vi "dataSave.vi"(8 "error in (no error)":errorcluster) -> (0 "error out":errorcluster)   [LabVIEW 2019]
uses:
  _ctrl/create-rw-close.ctl
  _ctrl/init-r-stop.ctl
  type-data.ctl
  _ctrl/rw.ctl
panel:
  out "# elements in queue":i32
  out "Numeric":i32
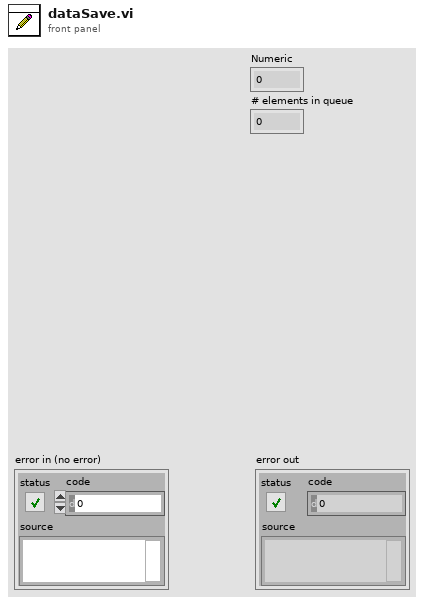
[diagram p1: front panel]
types:
  T1 = typedef "create-rw-close.ctl" = enum16{"create", "write", "read", "delete", "close"}
  T2 = typedef "init-r-stop.ctl" = enum16{"ini", "read", "stop"}
  T3 = typedef "type-data.ctl" = cluster{"dup path":path, "data":string}
  T4 = enum16{"open", "replace", "create", "open or create", "replace or create", "replace or create with confirmation"}
  T5 = typedef "rw.ctl" = enum16{"read", "write"}
  T6 = typedef "config_aging.ctl" = cluster{"Setting":T7, "TestName":string, "Result path":path, "파일 생성 주기[N]":u8, "Test Specs":T8}
  T7 = typedef "Setting_reg.ctl" = cluster{"제어 전압[V]":dbl, "출력전압[V]":dbl, "전류[A]":dbl, "출력전류[A]":dbl, "ON[초]":dbl, "OFF[초]":dbl, "Irms 허용치 from ":dbl, "Irms 허용치 to":dbl, "AO Delay ms":u32, "Log":path, "result":path}
  T8 = typedef "Breakdown-Spec.ctl" = cluster{"제어단 단선 Irms[mA](이하)":dbl, "제어단 특성 전류 Irms[mA] Max":dbl, "제어단 특성 전류 Irms[mA] Min":dbl, "출력단 단선 Irms[mA](이하)":dbl, "출력단 특성 전류 Irms[mA]  Max":dbl, "출력단 특성전류 Irms[mA]  Min":dbl, "온도[degree]":dbl}
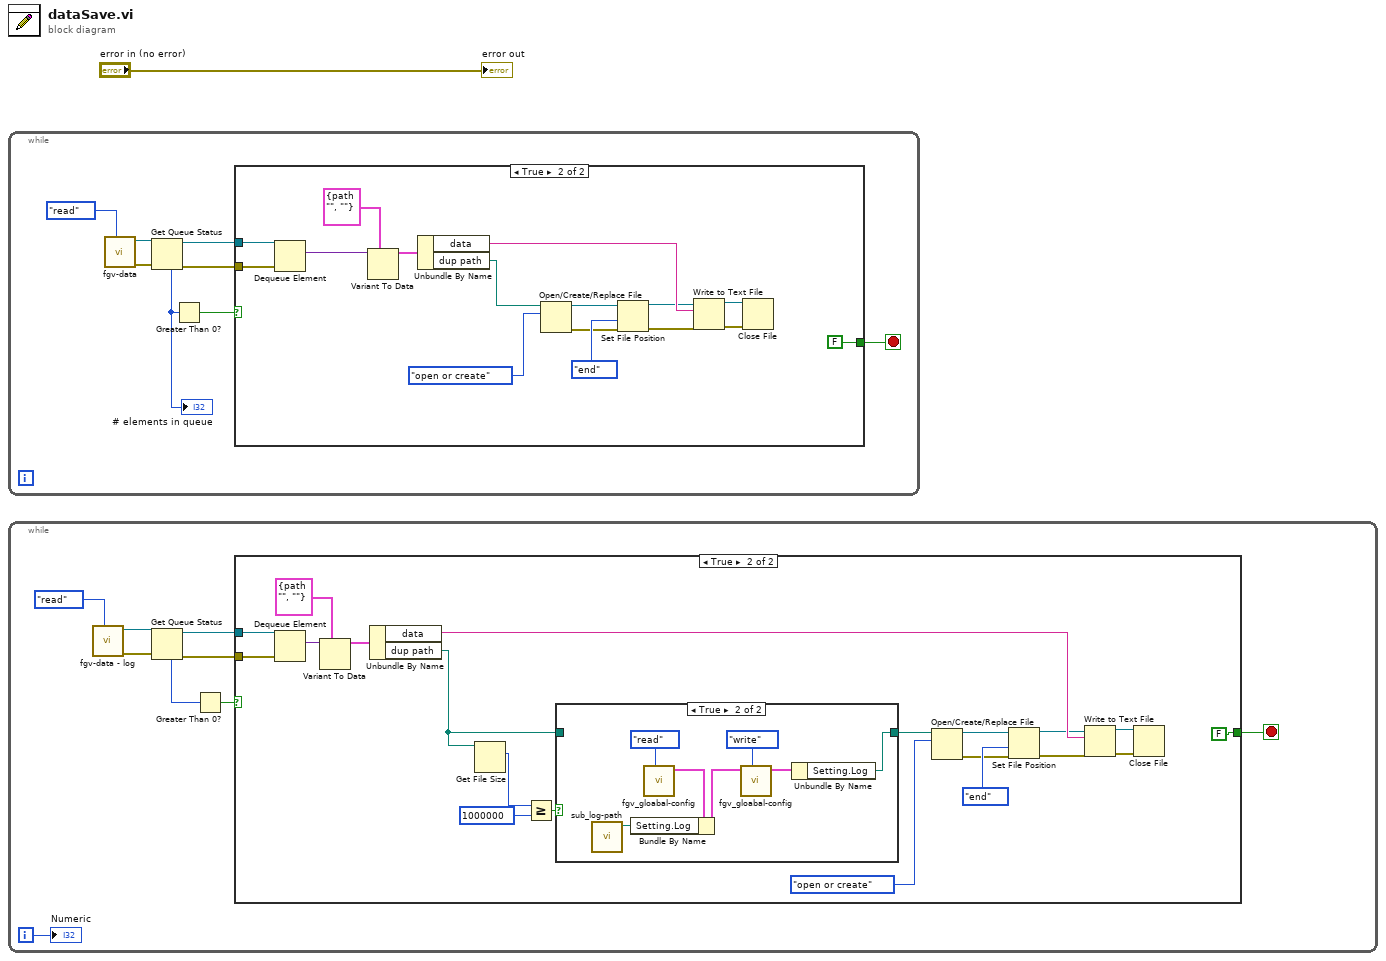
[diagram p0: block diagram]
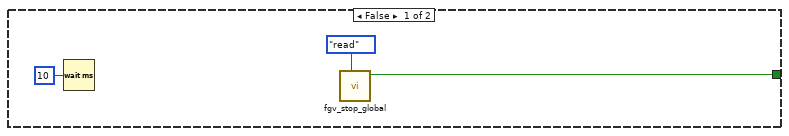
[diagram p2: hidden frame]
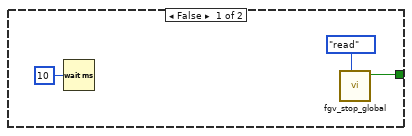
[diagram p4: hidden frame]
diagram:
  n1 = while {
    stop <- w3 stop-if-true
    n2 = call "fgv-data.vi"("cmd"=create-rw-close."read") -> ("error out"=w7:errorcluster, "queue out"=w8:refnum<queue>)  [unwired: 9 in]
    n3 = Get Queue Status(queue=w8, error in (no error)=w7) -> (queue out=w5:refnum<queue>, error out=w4:errorcluster, # elements in queue=w6:i32)  [unwired: 1 in, 5 out]
    "# elements in queue" <- w6
    n4 = Greater Than 0?(x=w6) -> (x > 0?=w2:bool)
    n5 = case shown="True" w2 {
      tunnel: w5 -> [_ w28]
      tunnel: w4 -> [_ w27]
      tunnel: [w11 FALSE] -> w3
      frame False {
        n6 = Wait (ms)(milliseconds to wait=u32 10) -> ()  [unwired: 1 out]
        n7 = call "fgv_stop_global.vi"("cmd"=init-r-stop."read") -> ("stop"=w11:bool)  [unwired: 10 in]
      }
      frame True {
        n8 = Dequeue Element(queue=w28, error in (no error)=w27) -> (element=w22:variant)  [unwired: 1 in, 3 out]
        n9 = Variant To Data(type=T3 {"dup path"=path "", "data"=""}, Variant=w22) -> (data=w20:T3)  [unwired: 1 in, 1 out]
        n10 = Unbundle By Name(w20) -> ("data"=w18:string, "dup path"=w19:path)
        n11 = Open/Create/Replace File(file path (use dialog)=w19, operation (0:open)=T4."open or create") -> (refnum out=w16:refnum<file>, error out=w14:errorcluster)  [unwired: 4 in, 1 out]
        n12 = Set File Position(refnum=w16, from (0:start)=enum16{"start", "end", "current"}."end", error in=w14) -> (refnum out=w15:refnum<file>, error out=w13:errorcluster)  [unwired: 1 in]
        n13 = Write to Text File(file (use dialog)=w15, text=w18, error in=w13) -> (refnum out=w25:refnum<file>, error out=w24:errorcluster)  [unwired: 1 in, 1 out]
        n14 = Close File(refnum=w25, error in=w24) -> ()  [unwired: 2 out]
      }
    }
  }
  n15 = while {
    i -> [w29]
    stop <- w34 stop-if-true
    n16 = call "fgv-data - log.vi"("cmd"=create-rw-close."read") -> ("error out"=w31:errorcluster, "queue out"=w32:refnum<queue>)  [unwired: 9 in]
    n17 = Get Queue Status(queue=w32, error in (no error)=w31) -> (queue out=w36:refnum<queue>, error out=w35:errorcluster, # elements in queue=w37:i32)  [unwired: 1 in, 5 out]
    n18 = Greater Than 0?(x=w37) -> (x > 0?=w30:bool)
    n19 = case shown="True" w30 {
      tunnel: w36 -> [_ w60]
      tunnel: w35 -> [_ w59]
      tunnel: [w39 FALSE] -> w34
      frame False {
        n20 = Wait (ms)(milliseconds to wait=u32 10) -> ()  [unwired: 1 out]
        n21 = call "fgv_stop_global.vi"("cmd"=init-r-stop."read") -> ("stop"=w39:bool)  [unwired: 10 in]
      }
      frame True {
        n22 = Dequeue Element(queue=w60, error in (no error)=w59) -> (element=w54:variant)  [unwired: 1 in, 3 out]
        n23 = Variant To Data(type=T3 {"dup path"=path "", "data"=""}, Variant=w54) -> (data=w52:T3)  [unwired: 1 in, 1 out]
        n24 = Unbundle By Name(w52) -> ("data"=w51:string, "dup path"=w41:path)
        n25 = Get File Size(file=w41) -> (size (in bytes)=w44:i64)  [unwired: 1 in, 2 out]
        n26 = Greater Or Equal?(x=w44, y=i64 1000000) -> (x >= y?=w45:bool)
        n27 = case shown="True" w45 {
          tunnel: [w61 w62] -> w42
          tunnel: w41 -> [w61 _]
          frame False {
          }
          frame True {
            n28 = call "sub_log-path.vi"() -> ("log path"=w64:path)  [unwired: 10 in, 1 out]
            n29 = call "fgv_gloabal-config.vi"("cmd"=rw."read") -> ("config_aging 2"=w67:T6)  [unwired: 10 in]
            n30 = Bundle By Name(cluster=w67, "Setting.Log"=w64) -> (w68:T6)
            n31 = call "fgv_gloabal-config.vi"("cmd"=rw."write", "config_aging"=w68) -> ("config_aging 2"=w63:T6)  [unwired: 9 in]
            n32 = Unbundle By Name(w63) -> ("Setting.Log"=w62:path)
          }
        }
        n33 = Open/Create/Replace File(file path (use dialog)=w42, operation (0:open)=T4."open or create") -> (refnum out=w49:refnum<file>, error out=w47:errorcluster)  [unwired: 4 in, 1 out]
        n34 = Set File Position(refnum=w49, from (0:start)=enum16{"start", "end", "current"}."end", error in=w47) -> (refnum out=w48:refnum<file>, error out=w46:errorcluster)  [unwired: 1 in]
        n35 = Write to Text File(file (use dialog)=w48, text=w51, error in=w46) -> (refnum out=w57:refnum<file>, error out=w56:errorcluster)  [unwired: 1 in, 1 out]
        n36 = Close File(refnum=w57, error in=w56) -> ()  [unwired: 2 out]
      }
    }
    "Numeric" <- w29
  }
  "error out" <- "error in (no error)"
